vi "EdgeRegistration and ObjectTracking.vi"() -> ()   [LabVIEW 2012]
uses:
  <vilib>/vision/NI_Vision_Development_Module.lvlib
panel:
  out "-x":dbl
  out "shift":T1(plugin-control)
  out "Objects 2":T2(array[cluster]) {"Aspect Ratio" format="%.2f"; "Orientation" format="%.2f"; "Area" format="%.2f"; "Object Center"."Y" format="%.2f"; "Object Center"."X" format="%.2f"}
  out "Objects":T2(array[cluster]) {"Aspect Ratio" format="%.2f"; "Orientation" format="%.2f"; "Area" format="%.2f"; "Object Center"."Y" format="%.2f"; "Object Center"."X" format="%.2f"}
  out "conv":T1(plugin-control)
  in  "Size & Tolerance 2":T3={"X Size"=3, "Y Size"=3, "% Tolerance"=40}
  in  "Settings 2":T4={"Objects"=0, "Threshold"=128, "Reject Border"=FALSE, "Fill Holes"=FALSE, "Min Object Size"=FALSE, "Min Size"=3, "Max Object Size"=FALSE, "Max Size"=100, "Show Search Area"=FALSE, "Show Center"=TRUE, "Show Bounding Box"=TRUE} {"Objects" items=["Bright Objects", "Dark Objects"]; "Threshold" min=1 max=999999999 step=1; "Max Size" min=1 max=999999999 step=1; "Min Size" min=1 max=999999999 step=1}
  out "Edge-detected 2":T1(plugin-control)
  out "Original Image 2":T1(plugin-control)
  in  "Filter Parameters 2":T5={"Sigma"=1.0, "HThresh"=0.7, "LThres"=0.2, "WindowSize"=9} {"LThres" min=0 max=1 format="%.2f"; "HThresh" min=0 max=1 format="%.2f"; "Sigma" min=0 max=1 format="%.2f"}
  in  "File Path 2":path
  in  "Size & Tolerance":T3={"X Size"=3, "Y Size"=3, "% Tolerance"=40}
  in  "Settings":T4={"Objects"=0, "Threshold"=128, "Reject Border"=FALSE, "Fill Holes"=FALSE, "Min Object Size"=FALSE, "Min Size"=3, "Max Object Size"=FALSE, "Max Size"=100, "Show Search Area"=FALSE, "Show Center"=TRUE, "Show Bounding Box"=TRUE} {"Objects" items=["Bright Objects", "Dark Objects"]; "Threshold" min=1 max=999999999 step=1; "Max Size" min=1 max=999999999 step=1; "Min Size" min=1 max=999999999 step=1}
  out "Edge-detected":T1(plugin-control)
  out "Original Image":T1(plugin-control)
  in  "Filter Parameters":T5={"Sigma"=1.0, "HThresh"=0.7, "LThres"=0.2, "WindowSize"=9} {"LThres" min=0 max=1 format="%.2f"; "HThresh" min=0 max=1 format="%.2f"; "Sigma" min=0 max=1 format="%.2f"}
  in  "File Path":path
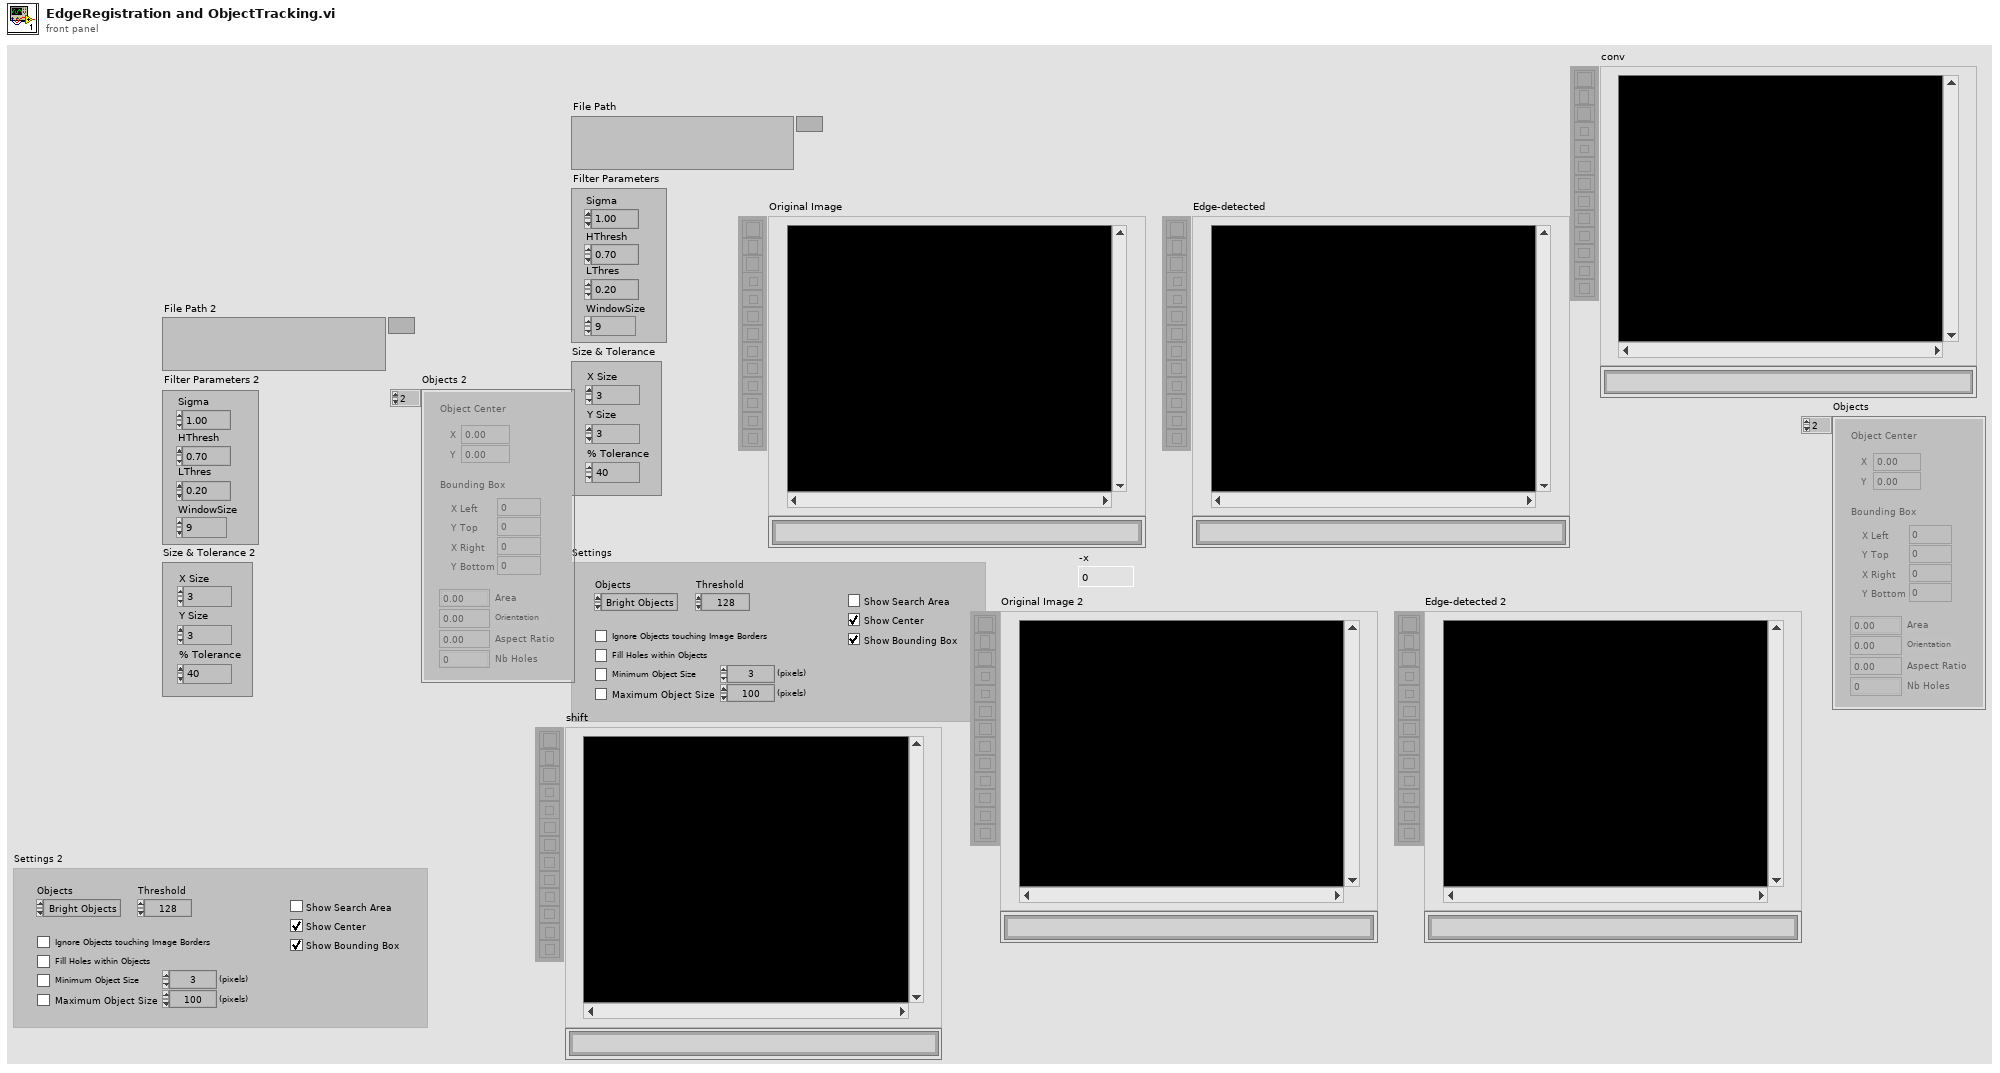
[diagram p1: front panel]
types:
  T1 = typedef "IMAQ Image.ctl" = refnum<image>
  T2 = cluster{"Object Center":cluster{"X":sgl, "Y":sgl}, "Bounding Box":cluster{"X Left":i32, "Y Top":i32, "X Right":i32, "Y Bottom":i32}, "Area":sgl, "Orientation":sgl, "Aspect Ratio":sgl, "Nb Holes":i32}[]
  T3 = cluster{"X Size":i32, "Y Size":i32, "% Tolerance":i32}
  T4 = cluster{"Objects":u16, "Threshold":i32, "Reject Border":bool, "Fill Holes":bool, "Min Object Size":bool, "Min Size":i32, "Max Object Size":bool, "Max Size":i32, "Show Search Area":bool, "Show Center":bool, "Show Bounding Box":bool}
  T5 = cluster{"Sigma":sgl, "HThresh":sgl, "LThres":sgl, "WindowSize":i32}
  T6 = typedef "Image Type" = u32
  T7 = enum32{"AutoM", "Close", "Dilate", "Erode", "Gradient", "Gradient in", "Gradient out", "HitMiss", "Open", "PClose", "POpen", "Thick", "Thin"}
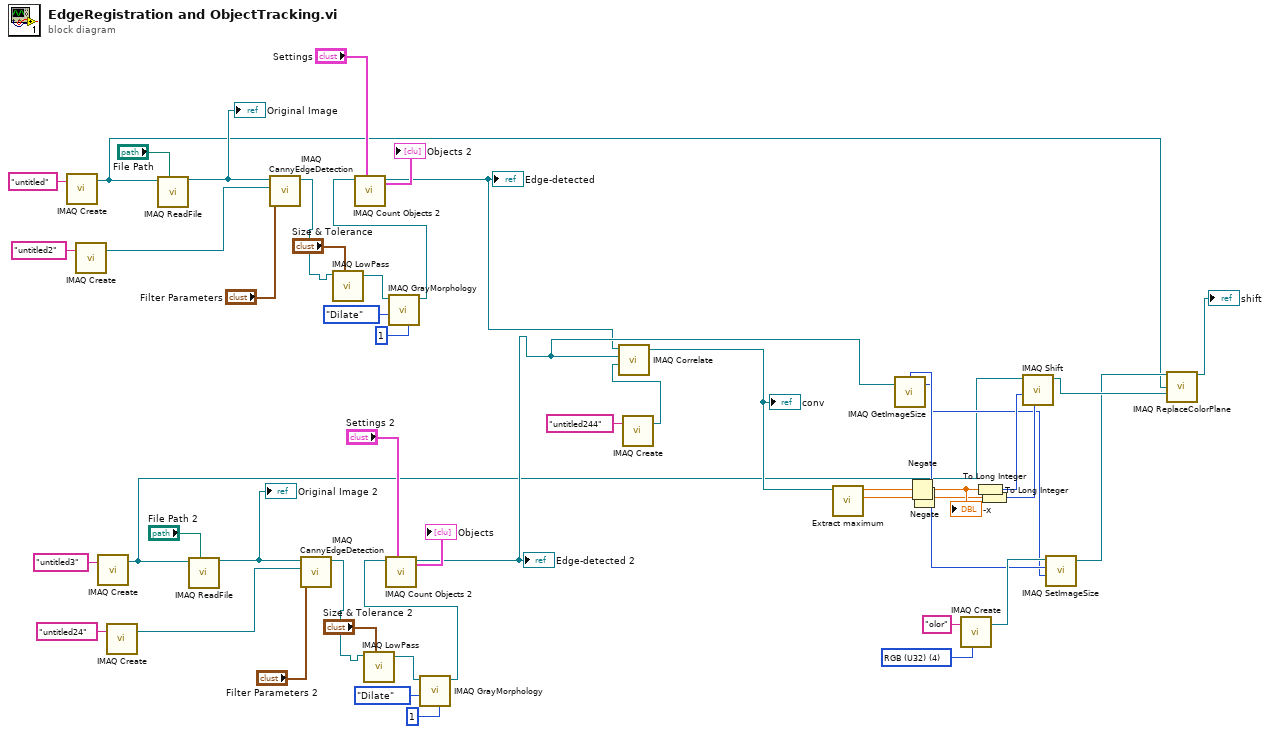
[diagram p0: block diagram]
diagram:
  w18 = T6 4 items=["Grayscale (U8)", "Grayscale (I16)", "Grayscale (SGL)", "Complex (CSG)", "RGB (U32)", "HSL (U32)", "RGB (U64)", "Grayscale (U16)"] ("Image Type")
  n1 = call "IMAQ Create"("Image Name"="untitled") -> ("New Image"=w3:T1)  [unwired: 4 in, 1 out]
  n2 = call "IMAQ Create"("Image Name"="untitled2") -> ("New Image"=w46:T1)  [unwired: 4 in, 1 out]
  n3 = call "IMAQ Create"("Image Name"="untitled3") -> ("New Image"=w4:T1)  [unwired: 4 in, 1 out]
  n4 = call "IMAQ Create"("Image Name"="untitled24") -> ("New Image"=w33:T1)  [unwired: 4 in, 1 out]
  n5 = call "IMAQ ReadFile"("File Path"="File Path", "Image"=w3) -> ("Image Out"=w44:T1)  [unwired: 5 in, 4 out]
  "Original Image" <- w44
  n6 = call "IMAQ ReadFile"("File Path"="File Path 2", "Image"=w4) -> ("Image Out"=w31:T1)  [unwired: 5 in, 4 out]
  "Original Image 2" <- w31
  n7 = call "IMAQ CannyEdgeDetection"("Image Src"=w44, "Image Dst"=w46, "Filter Parameters"="Filter Parameters") -> ("Image Dst Out"=w42:T1)  [unwired: 5 in, 1 out]
  n8 = call "IMAQ CannyEdgeDetection"("Image Src"=w31, "Image Dst"=w33, "Filter Parameters"="Filter Parameters 2") -> ("Image Dst Out"=w29:T1)  [unwired: 5 in, 1 out]
  n9 = call "IMAQ LowPass"("Image Src"=w42, "Size & Tolerance"="Size & Tolerance") -> ("Image Dst Out"=w38:T1)  [unwired: 5 in, 1 out]
  n10 = call "IMAQ LowPass"("Image Src"=w29, "Size & Tolerance"="Size & Tolerance 2") -> ("Image Dst Out"=w25:T1)  [unwired: 5 in, 1 out]
  n11 = call "IMAQ GrayMorphology"("Number of iterations (1)"=1, "Operation"=T7."Dilate", "Image Src"=w38) -> ("Image Dst Out"=w37:T1)  [unwired: 7 in, 1 out]
  n12 = call "IMAQ Count Objects 2"("Settings"="Settings", "Image"=w37) -> ("Image Out"=w11:T1, "Objects"=→"Objects 2":T2)  [unwired: 5 in, 3 out]
  "Edge-detected" <- w11
  n13 = call "IMAQ GrayMorphology"("Number of iterations (1)"=1, "Operation"=T7."Dilate", "Image Src"=w25) -> ("Image Dst Out"=w24:T1)  [unwired: 7 in, 1 out]
  n14 = call "IMAQ Count Objects 2"("Settings"="Settings 2", "Image"=w24) -> ("Image Out"=w15:T1, "Objects"=→"Objects":T2)  [unwired: 5 in, 3 out]
  "Edge-detected 2" <- w15
  n15 = call "IMAQ Create"("Image Name"="untitled244") -> ("New Image"=w22:T1)  [unwired: 4 in, 1 out]
  n16 = call "IMAQ Correlate"("Image Src"=w11, "Image Template"=w15, "Image Dst"=w22) -> ("Image Dst Out"=w16:T1)  [unwired: 4 in, 1 out]
  "conv" <- w16
  n17 = call "Extract maximum.vi"("Image in"=w16) -> ("y translation"=w13:dbl, "x translation"=w14:dbl)  [unwired: 7 in, 2 out]
  n18 = call "IMAQ GetImageSize"("Image"=w15) -> ("Y Resolution"=w5:i32, "X Resolution"=w6:i32)  [unwired: 3 in, 1 out]
  n19 = Negate(x=w14) -> (-x=w2:dbl)
  "-x" <- w2
  n20 = Negate(x=w13) -> (-x=w1:dbl)
  n21 = call "IMAQ Create"("Image Name"="olor", "Image Type"=w18) -> ("New Image"=w8:T1)  [unwired: 3 in, 1 out]
  n22 = To Long Integer(number=w2) -> (32bit integer=w10:i32)
  n23 = To Long Integer(number=w1) -> (32bit integer=w9:i32)
  n24 = call "IMAQ Shift"("YOffset"=w9, "XOffset"=w10, "Image Src"=w4) -> ("Image Dst Out"=w17:T1)  [unwired: 7 in, 1 out]
  n25 = call "IMAQ SetImageSize"("Y Resolution"=w5, "X Resolution"=w6, "Image"=w8) -> ("Image Out"=w7:T1)  [unwired: 2 in, 1 out]
  n26 = call "IMAQ ReplaceColorPlane"("Image Src"=w7, "Red or Hue Plane"=w3, "Green or Sat Plane"=w17) -> ("Image Dst Out"=→"shift":T1)  [unwired: 11 in, 1 out]
